vi "File handling - Run Number FGV.vi"(7 "Action(GET)":enum16{"GET", "SET"}(ring), 8 "error in (no error)":errorcluster, 10 "Run Status":T1) -> (0 "error out":errorcluster, 2 "Run Status":T1)   [LabVIEW 2011]
uses:
  Run Status Cluster.ctl
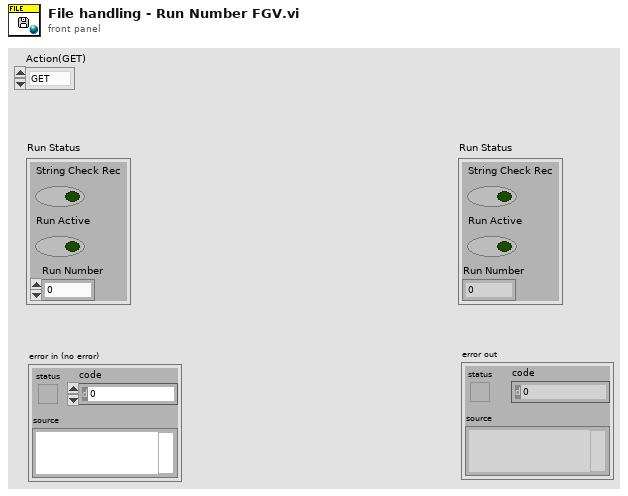
[diagram p1: front panel]
types:
  T1 = typedef "Run Status Cluster.ctl" = cluster{"String Check Rec":bool, "Run Active":bool, "Run Number":i32}
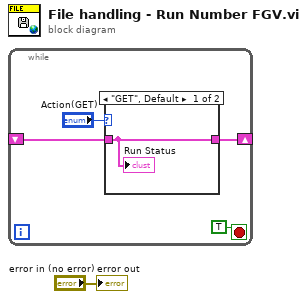
[diagram p0: block diagram]
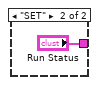
[diagram p2: hidden frame]
diagram:
  n1 = while {
    shift-right: [w2] -> _
    shift-left: _ -> [w3]
    stop <- TRUE stop-if-true
    n2 = case shown="\"GET\", Default" "Action(GET)" {
      tunnel: w3 -> [w6 _]
      tunnel: [w6 "Run Status"] -> w2
      frame "GET", Default {
        "Run Status" <- w6
      }
      frame "SET" {
      }
    }
  }
  "error out" <- "error in (no error)"
